vi "Mode_AE_V1.vi"(6 "Action":T1, 8 "Poke Mode In":dbl[][][](array[numeric]), 9 "Practical Mode In":dbl[][][](array[numeric]), 10 "Theoretical Mode In":dbl[][][](array[numeric])) -> (1 "Poke Mode Out":dbl[][][](array[numeric]), 2 "Practical Mode Out":dbl[][][](array[numeric]), 3 "Theoretical Mode Out":dbl[][][](array[numeric]))   [LabVIEW 2014]
uses:
  Controls/Standard Action.ctl
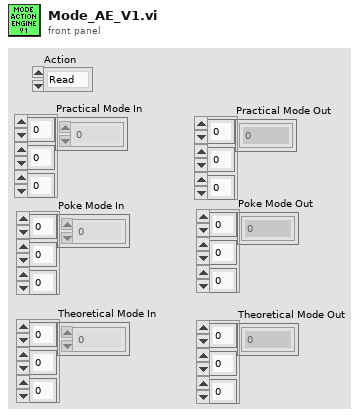
[diagram p1: front panel]
types:
  T1 = typedef "Standard Action.ctl" = enum16{"Read", "Write"}
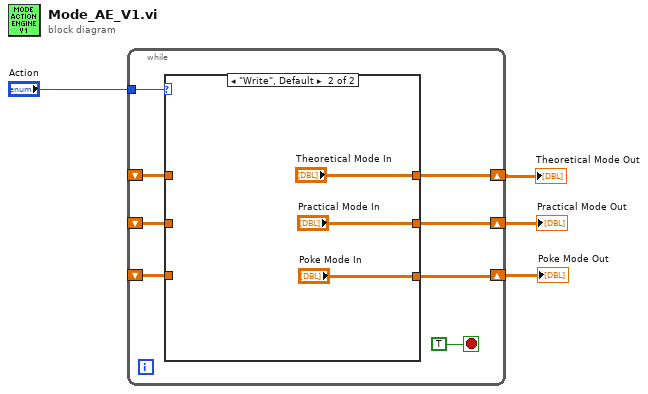
[diagram p0: block diagram]
diagram:
  n1 = while {
    tunnel: "Action" -> [w11]
    shift-right: [w10] -> w3
    shift-left: _ -> [w9]
    shift-right: [w8] -> w2
    shift-left: _ -> [w7]
    shift-right: [w6] -> w1
    shift-left: _ -> [w5]
    stop <- TRUE stop-if-true
    n2 = case shown="\"Write\", Default" w11 {
      tunnel: [w15 "Theoretical Mode In"] -> w10
      tunnel: w9 -> [w15 _]
      tunnel: [w14 "Practical Mode In"] -> w8
      tunnel: w7 -> [w14 _]
      tunnel: [w13 "Poke Mode In"] -> w6
      tunnel: w5 -> [w13 _]
      frame "Read" {
      }
      frame "Write", Default {
      }
    }
  }
  "Theoretical Mode Out" <- w3
  "Practical Mode Out" <- w2
  "Poke Mode Out" <- w1
